vi "HFRR ADV v022 new software.vi"() -> ()   [LabVIEW 2025] (continued)
            n3909 = Index Array(array=w5040, index #1=1 ("index")) -> (element #1=w5039:string, element #2=w5038:string, element #3=w5037:string, element #4=w5036:string, element #5=w5035:string, element #6=w5034:string)  [unwired: 5 in]
            n3910 = Index Array(array=w5030, index #1=1 ("index")) -> (element #1=w5029:string, element #2=w5028:string, element #3=w5027:string, element #4=w5026:string, element #5=w5025:string, element #6=w5024:string)  [unwired: 5 in]
            n3911 = Index Array(array=w5059, index #1=1 ("index")) -> (element #1=w5058:string, element #2=w5057:string, element #3=w5056:string, element #4=w5055:string, element #5=w5045:string, element #6=w5044:string)  [unwired: 5 in]
            n3912 = Index Array(array=w4979, index #1=1 ("index")) -> (element #1=w5011:string, element #2=w5010:string, element #3=w5009:string, element #4=w5008:string, element #5=w5007:string, element #6=w5006:string)  [unwired: 5 in]
            n3913 = local read "SEN.RUN HRS"() -> (w4982:dbl)
            n3914 = Divide(x=w4986, y=w4994) -> (x/y=w4993:dbl)
            n3915 = Increment(x=w4993) -> (x+1=w4989:dbl)
            n3916 = Number To Decimal String(number=w4989) -> (decimal integer string=→"run hrs":string)  [unwired: 1 in]
            n3917 = Divide(x=w4982, y=3600.0 ("f")) -> (x/y=w4977:dbl)
            n3918 = Round To Nearest(number=w4977) -> (nearest integer value=w4975:dbl)
            n3919 = Number To Decimal String(number=w4975) -> (decimal integer string=w4976:string)  [unwired: 1 in]
            n3920 = Number To Decimal String(number=w4984) -> (decimal integer string=w4985:string)  [unwired: 1 in]
            n3921 = local read "Model No"() -> (w4990:string)
            n3922 = local read "UUID"() -> (w5085:string)
            n3923 = local read "Serial No"() -> (w5089:string)
            n3924 = local read "Secret Key"() -> (w5090:string)
            n3925 = Concatenate Strings("\",\"MachineSerialNumber\":\"" ("string"), w5089) -> (w5093:string)
            n3926 = Concatenate Strings("\",\"ModelNumber\":\"" ("string"), w4990) -> (w4991:string)
            n3927 = Concatenate Strings("\",\"MachineRuntimeHours\":\"" ("string"), w4976) -> (w5094:string)
            n3928 = Concatenate Strings("\",\"MachineRuntimeCycles\":\"", w4985) -> (w5087:string)
            n3929 = Concatenate Strings(w5043, w5039) -> (w5073:string)
            n3930 = Concatenate Strings(w5042, w5029) -> (w5074:string)
            n3931 = Concatenate Strings(w5041, w5011) -> (w5072:string)
            n3932 = Concatenate Strings(w5093, w4991, w5094, w5087) -> (w5096:string)
            n3933 = Concatenate Strings(w5043, w5038) -> (w5070:string)
            n3934 = Concatenate Strings(w5042, w5028) -> (w5069:string)
            n3935 = Concatenate Strings(w5041, w5010) -> (w5071:string)
            n3936 = Concatenate Strings(w5043, w5037) -> (w5065:string)
            n3937 = Concatenate Strings(w5042, w5027) -> (w5066:string)
            n3938 = Concatenate Strings(w5041, w5009) -> (w5064:string)
            n3939 = Concatenate Strings(w5043, w5036) -> (w5062:string)
            n3940 = Concatenate Strings(w5042, w5026) -> (w5061:string)
            n3941 = Concatenate Strings(w5041, w5008) -> (w5063:string)
            n3942 = Concatenate Strings(w5073, w5074, w5072) -> (w5075:string)
            n3943 = Concatenate Strings(w5043, w5035) -> (w5052:string)
            n3944 = Concatenate Strings(w5042, w5025) -> (w5053:string)
            n3945 = Concatenate Strings(w5043, w5034) -> (w5049:string)
            n3946 = Concatenate Strings(w5042, w5024) -> (w5048:string)
            n3947 = Concatenate Strings(w5041, w5007) -> (w5051:string)
            n3948 = Concatenate Strings(w5041, w5006) -> (w5050:string)
            n3949 = Concatenate Strings("{\"SecretKey\":\"", w5090, w5096, "\",\"UUID\" : \"", w5085, "\",\"SensorInformation\":", "[{" ("string")) -> (w5023:string)
            n3950 = Concatenate Strings(w5070, w5069, w5071) -> (w5068:string)
            n3951 = Concatenate Strings(w5065, w5066, w5064) -> (w5067:string)
            n3952 = Concatenate Strings(w5062, w5061, w5063) -> (w5060:string)
            n3953 = Concatenate Strings(w5052, w5053, w5051) -> (w5054:string)
            n3954 = Concatenate Strings(w5049, w5048, w5050) -> (w5047:string)
            n3955 = Concatenate Strings(w5046, w5058, w5075, w5016) -> (w5022:string)
            n3956 = Concatenate Strings(w5046, w5057, w5068, w5016) -> (w5021:string)
            n3957 = Concatenate Strings(w5046, w5056, w5067, w5016) -> (w5020:string)
            n3958 = Concatenate Strings(w5046, w5055, w5060, w5016) -> (w5019:string)
            n3959 = Concatenate Strings(w5046, w5045, w5054, w5016) -> (w5018:string)
            n3960 = Concatenate Strings(w5046, w5044, w5047, "\"}" ("string")) -> (w5017:string)
            n3961 = Concatenate Strings(w5023, w5022, w5021, w5020, w5019, w5018, w5017, "]}" ("string")) -> (w5014:string)
            n3962 = local read "SEN.RUN HRS"() -> (w4981:dbl)
            n3963 = disable-structure shown="Disabled" {
              frame Disabled {
                n3964 = local read "state"() -> (w5100:string[])
                n3965 = Delete From Array(array=w5100, index=0) -> (array with subset deleted=w5098:string[])  [unwired: 1 in, 1 out]
                n3966 = for {
                  N: 6 -> [_]
                  tunnel: w5098 -> [w5111] mode=indexing
                  tunnel: [w5110] -> w5097 mode=indexing
                  n3967 = Equal?(x=w5111, y="Warning") -> (x = y?=w5107:bool)
                  n3968 = Equal?(x=w5111, y="Healthy") -> (x = y?=w5104:bool)
                  n3969 = Select(t="2" ("y"), s=w5107, f="3" ("y")) -> (s? t:f=w5102:string)
                  n3970 = Select(t="1" ("y"), s=w5104, f=w5102) -> (s? t:f=w5110:string)
                }
                "state1" <- w5097
              }
              frame Enabled {
              }
            }
            n3971 = stacked-sequence {
              tunnel: w5014 -> [w5122 _ _]
              tunnel: [_ _ w5138] -> _
              frame #0 {
                (unwired) FALSE ("convert eol (F)")
                w5124 = enum16{"start", "end", "current"}."start" ("pos mode (0:2)")
                n3972 = local read "Path"() -> (w5118:path)
                n3973 = Path To String(path=w5118) -> (string=w5130:string)
                n3974 = Concatenate Strings(w5130, "\\", "Sensor File Name") -> (w5131:string)
                n3975 = local write "standard output 2"(" ") -> ()
                n3976 = String To Path(string=w5131) -> (path=w5121:path)
                n3977 = call <vilib>:"Open_Create_Replace File.vi"("advisory dialog? (display:T)"=FALSE, "function (open:0)"=T32."create or replace", "file path"=w5121) -> ("error out"=w5134:errorcluster, "refnum"=w5133:refnum<file>)  [unwired: 5 in, 2 out]
                n3978 = Set File Position(refnum=w5133, from (0:start)=w5124, error in=w5134) -> (refnum out=w5114:refnum<file>, error out=w5113:errorcluster)  [unwired: 1 in]
                n3979 = Write to Binary File(file (use dialog)=w5114, data=" ", error in=w5113, 5:FALSE ("prepend array or string size? (T)")) -> (refnum out=w5125:refnum<file>, error out=w5126:errorcluster)  [unwired: 2 in, 1 out]
                n3980 = Set File Position(offset (in bytes) (0)=w5124, refnum=w5125, error in=w5126) -> (refnum out=w5117:refnum<file>, error out=w5116:errorcluster)  [unwired: 1 in]
                n3981 = Write to Binary File(file (use dialog)=w5117, data=w5122, error in=w5116, 5:FALSE ("prepend array or string size? (T)")) -> (error out=w5120:errorcluster)  [unwired: 2 in, 2 out]
                n3982 = flat-sequence {
                  tunnel: w5121 -> [w5136]
                  tunnel: w5120 -> [_]
                  frame #0 {
                    n3983 = call <vilib>:"Read Characters From File.vi"("file path (dialog if empty)"=w5136) -> ("character string"=→"Sensor Health JSON string":string)  [unwired: 5 in, 3 out]
                  }
                }
                "SinglePoint  2" <- w5122
              }
              frame #1 {
              }
              frame #2 {
                (unwired) "\"Stored\": true" ("string")
                n3984 = call <vilib>:"System Exec.vi"("run minimized? (F)"=TRUE, "wait until completion? (T)"=TRUE, "working directory"=path "C:/LAB-IQ-NXT", "command line"="C:\\LAB-IQ-NXT\\JPostH.bat") -> ("standard error"=→"Respose From Server 2":string, "standard output"=w5141:string)  [unwired: 4 in, 2 out]
                "standard output 2" <- w5141
                n3985 = Match Pattern(string=w5141, regular expression="JSONH Check String") -> (match substring=w5139:string, offset past match=w5138:i32)  [unwired: 1 in, 2 out]
                n3986 = Equal?(x=w5139, y="JSONH Check String") -> (x = y?=→"Upload \nConfirmed 2":bool)
              }
            }
            n3987 = Divide(x=w4981, y=3600.0 ("f")) -> (x/y=w4974:dbl)
            n3988 = local read "run time"() -> (w5031:string[])
            n3989 = Round To Nearest(number=w4974) -> (nearest integer value=w4973:dbl)
            n3990 = Number To Decimal String(number=w4973) -> (decimal integer string=w4972:string)  [unwired: 1 in]
            n3991 = Index Array(array="Sensor Information", index (col) #1=0 ("disabled index (col)"), index (col) #2=1 ("index (col)"), index (col) #3=2 ("index (col)"), index (col) #4=3 ("index (col)")) -> (element #1=→"Sensor name":string[], element #2=→"model num":string[], element #3=→"run time":string[], element #4=→"state":string[])  [unwired: 4 in]
            n3992 = Insert Into Array(array=w5031, index=1, new element #1=w4972, new element #2=w4972, new element #3=w4972, new element #4=w4972, new element #5=w4972, new element #6=w4972) -> (w4996:string[])
            "run" <- w4996
            n3993 = local read "out"() -> (w4978:string[])
            n3994 = local read "Sensor Information"() -> (w4998:string[][])
            n3995 = Replace Array Subset(array=w4998, new element #1=w4996, index (col) #1=2 ("disabled index (col)"), new element #2=w4978, index (col) #2=3 ("index (col)")) -> (w4997:string[][])  [unwired: 2 in]
            n3996 = local write "Sensor Information"(w4997) -> ()
          }
        }
        n3997 = case shown="True" w4945 {
          frame False {
          }
          frame True {
            n3998 = Equal?(x="FLAG", y=0.0) -> (x = y?=w4962:bool)
            n3999 = case shown="False" w4962 {
              frame False {
                n4000 = Get Date/Time In Seconds() -> (seconds since 1Jan1904=w4968:timestamp)
                n4001 = local read "START 2"() -> (w4966:dbl)
                n4002 = To Double Precision Float(number=w4968) -> (double precision float=w4967:dbl)
                n4003 = Subtract(x=w4967, y=w4966) -> (x-y=→"SENSOR TIME  2":dbl)
              }
              frame True {
                n4004 = Get Date/Time In Seconds() -> (seconds since 1Jan1904=w4970:timestamp)
                n4005 = To Double Precision Float(number=w4970) -> (double precision float=→"START 2":dbl)
                n4006 = local write "FLAG"(100.0 ("FLAG")) -> ()
              }
            }
          }
        }
        n4007 = disable-structure shown="Disabled" {
          disable-tunnel: w4948 -> [w4957 _]
          disable-tunnel: [w4956 _] -> w4947
          frame Disabled {
            n4008 = local read "Json St Flg"() -> (w4955:bool)
            n4009 = case shown="True" w4955 {
              tunnel: w4957 -> [w4958 w4960]
              tunnel: [w4958 w4959] -> w4956
              frame False {
              }
              frame True {
                n4010 = Increment(x=w4960) -> (x+1=w4959:dbl)
                "T cycle" <- w4959
                n4011 = local write "Json St Flg"(FALSE ("Json St Flg")) -> ()
              }
            }
          }
          frame Enabled {
          }
        }
        n4012 = local read "Quit"() -> (w4942:bool)
      }
    }
    frame Enabled {
    }
  }
  n4013 = stacked-sequence {
    tunnel: [w5340] -> w44
    frame #0 {
      w5340 = FALSE ("Upload \nConfirmed")
      n4014 = local write "Upload \nConfirmed"(w5340) -> ()
      n4015 = local write "St Str"("") -> ()
    }
  }
  n4016 = disable-structure shown="Disabled" {
    disable-tunnel: w44 -> [w5341 _]
    frame Disabled {
      n4017 = case shown="True" {
        selector: _ -> [_ _]
        tunnel: w5341 -> [_ w5342]
        frame False {
        }
        frame True {
          n4018 = while {
            tunnel: [w5348] -> _
            tunnel: w5342 -> [_]
            i -> [w5348]
            stop <- w5343 stop-if-true
            n4019 = local read "Json End Flg"() -> (w5347:bool)
            n4020 = Wait (ms)(milliseconds to wait=u32 20 ("Refresh Rate (ms)")) -> ()  [unwired: 1 out]
            n4021 = local read "refresh flag"() -> (w5344:bool)
            n4022 = local read "RUN"() -> (w5345:bool)
            n4023 = And(x=w5345, y=w5344) -> (x .and. y?=w5346:bool)
            n4024 = Or(x=w5346, y=w5347) -> (x .or. y?=w5349:bool)
            "AR Led" <- w5349
            n4025 = case shown="True" w5349 {
              frame False {
              }
              frame True {
                w5366 = "\",\""
                n4026 = local read "UUID"() -> (w5364:string)
                n4027 = local write "refresh flag"(FALSE ("refresh flag")) -> ()
                n4028 = local read "time"() -> (w5353:dbl)
                n4029 = Multiply(x=w5353, y=60.0) -> (x*y=w5352:dbl)
                n4030 = Concatenate Strings("UUID\" : \"", w5364, "\"}") -> (w5367:string)
                n4031 = Number To Fractional String(number=w5352, width (-)=i16 10, precision (6)=i16 4) -> (F-format string=w5381:string)  [unwired: 1 in]
                n4032 = Concatenate Strings("{", "\"Time\":\"", w5381, w5366) -> (w5376:string)
                n4033 = stacked-sequence {
                  tunnel: w5366 -> [w5429 w5437 w5444 w5452 w5460 w5469 w5476]
                  tunnel: [w5430 _ _ _ _ _ _] -> w5380
                  tunnel: [_ w5438 _ _ _ _ _] -> w5379
                  tunnel: [_ _ w5445 _ _ _ _] -> w5378
                  tunnel: [_ _ _ w5454 _ _ _] -> w5377
                  tunnel: w5367 -> [_ _ _ _ _ _ w5487]
                  tunnel: [_ _ _ _ _ _ w5486] -> w5363
                  tunnel: [_ _ _ _ _ w5466 _] -> w5362
                  tunnel: [_ _ _ _ w5459 _ _] -> w5361
                  frame #0 {
                    n4034 = local read "NORMAL LOAD"() -> (w5428:dbl)
                    n4035 = Number To Fractional String(number=w5428, width (-)=i16 10, precision (6)=i16 4) -> (F-format string=w5431:string)  [unwired: 1 in]
                    n4036 = Concatenate Strings("NormalLoad\":\"", w5431, w5429) -> (w5430:string)
                  }
                  frame #1 {
                    n4037 = local read "Temp"() -> (w5436:dbl)
                    n4038 = Number To Fractional String(number=w5436, width (-)=i16 10, precision (6)=i16 4) -> (F-format string=w5439:string)  [unwired: 1 in]
                    n4039 = Concatenate Strings("Temperature\":\"", w5439, w5437) -> (w5438:string)
                  }
                  frame #2 {
                    n4040 = local read "cof"() -> (w5442:dbl)
                    n4041 = Number To Fractional String(number=w5442, width (-)=i16 10, precision (6)=i16 4) -> (F-format string=w5446:string)  [unwired: 1 in]
                    n4042 = Concatenate Strings("FrictionalForce\":\"", w5446, w5444) -> (w5445:string)
                  }
                  frame #3 {
                    n4043 = local read "Set Hz"() -> (w5450:dbl)
                    n4044 = Multiply(x=w5450, y=60.0) -> (x*y=w5449:dbl)
                    n4045 = Number To Fractional String(number=w5449, width (-)=i16 10, precision (6)=i16 4) -> (F-format string=w5455:string)  [unwired: 1 in]
                    n4046 = Concatenate Strings("Speed\":\"", w5455, w5452) -> (w5454:string)
                  }
                  frame #4 {
                    n4047 = local read item#-1() -> (w5458)
                    n4048 = Number To Fractional String(number=w5458, width (-)=i16 10, precision (6)=i16 4) -> (F-format string=w5462:string)  [unwired: 1 in]
                    n4049 = Concatenate Strings("LinearDeformation\":\"", w5462, w5460) -> (w5459:string)
                  }
                  frame #5 {
                    n4050 = local read "AIR TEMP"() -> (w5465:dbl)
                    n4051 = local read "Json St Flg"() -> (w5467:bool)
                    n4052 = local read "Json End Flg"() -> (w5468:bool)
                    n4053 = Number To Fractional String(number=w5465, width (-)=i16 10, precision (6)=i16 4) -> (F-format string=w5471:string)  [unwired: 1 in]
                    n4054 = Concatenate Strings("Vibration\":\"", w5471, w5469) -> (w5466:string)
                    n4055 = And(x=w5467, y=w5468) -> ()  [unwired: 1 out]
                  }
                  frame #6 {
                    n4056 = local read "Json End Flg"() -> (w5475:bool)
                    n4057 = Get Date/Time In Seconds() -> (seconds since 1Jan1904=w5483:timestamp)
                    n4058 = local read "Json St Flg"() -> (w5474:bool)
                    n4059 = To Double Precision Float(number=w5483) -> (double precision float=w5482:dbl)
                    n4060 = Subtract(x=w5482, y=2082844800.0) -> (x-y=w5480:dbl)
                    n4061 = Number To Fractional String(number=w5480, width (-)=i16 12, precision (6)=i16 0) -> (F-format string=w5477:string)  [unwired: 1 in]
                    n4062 = case shown="True" w5475 {
                      tunnel: ["" w5490] -> w5484
                      tunnel: w5477 -> [_ w5491]
                      tunnel: w5476 -> [_ w5489]
                      frame False {
                      }
                      frame True {
                        n4063 = local write "Json End Flg"(FALSE ("Json St Flg")) -> ()
                        n4064 = Concatenate Strings("End\": \"", w5491, w5489) -> (w5490:string)
                      }
                    }
                    n4065 = case shown="True" w5474 {
                      tunnel: [w5494 w5497] -> w5485
                      tunnel: w5477 -> [_ w5498]
                      tunnel: w5476 -> [_ w5495]
                      frame False {
                        n4066 = local read "St Str"() -> (w5494:string)
                      }
                      frame True {
                        n4067 = Concatenate Strings("Start\":\"", w5498, w5495) -> (w5497:string)
                        "St Str" <- w5497
                        n4068 = local write "Json St Flg"(FALSE ("Json St Flg")) -> ()
                      }
                    }
                    n4069 = Concatenate Strings(w5485, w5484, w5487) -> (w5486:string)
                  }
                }
                n4070 = local read "FILE"() -> (w5355:string)
                n4071 = Concatenate Strings("\",\"OperatorID\":\"" ("string"), "Operator ID") -> (w5358:string)
                n4072 = Concatenate Strings("\",\"DatasetTitle\":\"" ("string"), w5355) -> (w5357:string)
                n4073 = Concatenate Strings("\",\"SerialNumber\":\"" ("string"), "Serial No") -> (w5387:string)
                n4074 = Concatenate Strings("\",\"ModelNumber\":\"" ("string"), "Model No") -> (w5386:string)
                n4075 = Concatenate Strings(w5387, w5386) -> (w5369:string)
                n4076 = Concatenate Strings("{\"SecretKey\":\"", "Secret Key", w5369, w5358, w5357, "\",\"Samples\":[") -> (w5374:string)
                n4077 = Concatenate Strings(w5376, w5380, w5379, w5378, w5377, w5361, w5362, w5363) -> (w5375:string)
                n4078 = Concatenate Strings(w5374, w5375, "]}") -> (w5373:string)
                n4079 = stacked-sequence {
                  tunnel: w5373 -> [w5402 _ _]
                  tunnel: [_ _ w5419] -> _
                  frame #0 {
                    (unwired) FALSE ("convert eol (F)")
                    w5404 = enum16{"start", "end", "current"}."start" ("pos mode (0:2)")
                    n4080 = Path To String(path="Path") -> (string=w5410:string)
                    n4081 = Concatenate Strings(w5410, "\\", "Data File Name") -> (w5412:string)
                    n4082 = local write "standard output"(" ") -> ()
                    n4083 = String To Path(string=w5412) -> (path=w5401:path)
                    n4084 = call <vilib>:"Open_Create_Replace File.vi"("advisory dialog? (display:T)"=FALSE, "function (open:0)"=T32."create or replace", "file path"=w5401) -> ("error out"=w5415:errorcluster, "refnum"=w5414:refnum<file>)  [unwired: 5 in, 2 out]
                    n4085 = Set File Position(refnum=w5414, from (0:start)=w5404, error in=w5415) -> (refnum out=w5395:refnum<file>, error out=w5394:errorcluster)  [unwired: 1 in]
                    n4086 = Write to Binary File(file (use dialog)=w5395, data=" ", error in=w5394, 5:FALSE ("prepend array or string size? (T)")) -> (refnum out=w5405:refnum<file>, error out=w5406:errorcluster)  [unwired: 2 in, 1 out]
                    n4087 = Set File Position(offset (in bytes) (0)=w5404, refnum=w5405, error in=w5406) -> (refnum out=w5398:refnum<file>, error out=w5397:errorcluster)  [unwired: 1 in]
                    n4088 = Write to Binary File(file (use dialog)=w5398, data=w5402, error in=w5397, 5:FALSE ("prepend array or string size? (T)")) -> (error out=w5400:errorcluster)  [unwired: 2 in, 2 out]
                    n4089 = flat-sequence {
                      tunnel: w5401 -> [w5417]
                      tunnel: w5400 -> [_]
                      frame #0 {
                        n4090 = call <vilib>:"Read Characters From File.vi"("file path (dialog if empty)"=w5417) -> ("character string"=→"JSON string":string)  [unwired: 5 in, 3 out]
                      }
                    }
                    "SinglePoint" <- w5402
                  }
                  frame #1 {
                  }
                  frame #2 {
                    (unwired) "\"Stored\": true" ("string")
                    n4091 = call <vilib>:"System Exec.vi"("run minimized? (F)"=TRUE, "wait until completion? (T)"=TRUE, "working directory"=path "C:/LAB-IQ-NXT", "command line"="C:\\LAB-IQ-NXT\\JPost.bat") -> ("standard error"=→"Respose From Server":string, "standard output"=w5422:string)  [unwired: 4 in, 2 out]
                    "standard output" <- w5422
                    n4092 = Match Pattern(string=w5422, regular expression="JSON Check String") -> (match substring=w5420:string, offset past match=w5419:i32)  [unwired: 1 in, 2 out]
                    n4093 = Equal?(x=w5420, y="JSON Check String") -> (x = y?=→"Upload \nConfirmed":bool)
                  }
                }
              }
            }
            n4094 = local read "Quit"() -> (w5343:bool)
          }
        }
      }
    }
    frame Enabled {
    }
  }
  n4095 = disable-structure shown="Disabled" {
    disable-tunnel: _ -> [w5505 _]
    frame Disabled {
      n4096 = while {
        shift-right: [w5513] -> w5501
        shift-left: _ -> [w5514]
        shift-right: [w5511] -> w5502
        shift-left: errorcluster {"status"=TRUE, "code"=0, "source"="Init"} ("error out") -> [w5512]
        shift-right: [w5509] -> _
        shift-left: "" -> [w5510]
        tunnel: [w5507] -> _
        tunnel: w5505 -> [_]
        i -> [w5507]
        stop <- w5506 stop-if-true
        n4097 = flat-sequence {
          tunnel: [w5515] -> w5508
          frame #0 {
            n4098 = Wait (ms)(milliseconds to wait=10.0 ("Delay")) -> (millisecond timer value=w5515:u32)
          }
        }
        n4099 = case shown="No Error" w5512 {
          selector: w5512 -> [w5545 w5664]
          tunnel: [w5528 w5666] -> w5513
          tunnel: [w5527 w5665] -> w5511
          tunnel: w5514 -> [w5546 w5658]
          tunnel: w5510 -> [w5526 w5657]
          tunnel: [w5525 w5657] -> w5509
          tunnel: w5508 -> [_ _]
          frame No Error {
            n4100 = Concatenate Strings("\r", "\n") -> (w5537:string)  [unwired: 1 in]
            n4101 = case shown="True" w5538 {
              tunnel: w5546 -> [w5570 w5577]
              tunnel: w5545 -> [w5569 w5576]
              tunnel: [w5570 w5575] -> w5544
              tunnel: [w5569 w5574] -> w5524
              tunnel: w5537 -> [_ w5573]
              frame False {
              }
              frame True {
                n4102 = VISA Write(VISA resource name=w5577, write buffer=w5573, error in (no error)=w5576) -> (VISA resource name out=w5575:refnum<visa-resource-name>, error out=w5574:errorcluster)  [unwired: 1 out]
                n4103 = local write "Read String"("") -> ()
                n4104 = local write item#-1(FALSE) -> ()
              }
            }
            n4105 = property class="Instr"(reference=w5544, error in=w5524) -> (reference out=w5543:refnum<visa-resource-name>, error out=w5542:errorcluster, "Serial Settings:Number of Bytes at Serial Port"=w5541:u32)
            n4106 = Greater?(x=w5541, y=u32 100) -> (0:w5539:bool)
            n4107 = case shown="True" w5539 {
              tunnel: w5543 -> [w5580 w5604]
              tunnel: w5542 -> [w5579 w5603]
              tunnel: w5541 -> [_ w5602]
              tunnel: [w5580 w5601] -> w5530
              tunnel: [w5579 w5600] -> w5529
              tunnel: w5526 -> [w5578 w5599]
              tunnel: [w5578 ""] -> w5525
              frame False {
              }
              frame True {
                w5589 = u32 6 ("y")
                # "Page 84 of \nmanual"
                n4108 = VISA Read(VISA resource name=w5604, byte count=w5602, error in (no error)=w5603) -> (VISA resource name out=w5601:refnum<visa-resource-name>, read buffer=w5597:string, error out=w5600:errorcluster)  [unwired: 1 out]
                n4109 = while {
                  tunnel: w5597 -> [w5653]
                  tunnel: [w5649] -> w5591 mode=indexing
                  tunnel: [w5643] -> w5595 mode=indexing
                  tunnel: [w5641] -> _
                  i -> [w5641]
                  stop <- w5646 stop-if-true
                  n4110 = String Subset(string=w5653, offset (0)=w5641) -> (substring=w5648:string)  [unwired: 1 in]
                  n4111 = String To Byte Array(string=w5648) -> (unsigned byte array=w5652:u8[])
                  n4112 = String Length(string=w5648) -> (length=w5647:i32)
                  n4113 = Index Array(array=w5652) -> (element=w5651:u8)  [unwired: 1 in]
                  n4114 = Equal To 0?(x=w5647) -> (x = 0?=w5646:bool)
                  n4115 = Number To Boolean Array(number=w5651) -> (Boolean array=w5645:bool[])
                  n4116 = Reverse 1D Array(array=w5645) -> (reversed array=w5644:bool[])
                  n4117 = And(x=w5645, y=bool[] [FALSE, FALSE, FALSE, FALSE, FALSE, FALSE, TRUE, TRUE] ("Boolean array")) -> (x .and. y?=w5649:bool[])
                  n4118 = And(x=w5644, y=bool[] [FALSE, FALSE, TRUE, TRUE, TRUE, TRUE, TRUE, TRUE] ("Boolean array")) -> (x .and. y?=w5643:bool[])
                }
                n4119 = Concatenate Strings(w5599, w5597) -> (→"Read String":string)
                n4120 = while {
                  tunnel: w5591 -> [w5640] mode=indexing
                  tunnel: [w5636] -> w5594
                  i -> [w5636]
                  stop <- w5637 stop-if-true
                  n4121 = Search 1D Array(1D array=w5640, element=TRUE) -> (index of element=w5638:i32)  [unwired: 1 in]
                  n4122 = Less Than 0?(x=w5638) -> (x < 0?=w5637:bool)
                }
                n4123 = Delete From Array(array=w5595, length=w5594, index (row)=0) -> (array with subset deleted=w5590:bool[][])  [unwired: 1 in, 1 out]
                n4124 = Array Size(array=w5590) -> (size(s)=w5592:i32[])
                n4125 = Index Array(array=w5592) -> (element=w5584:i32)  [unwired: 1 in]
                n4126 = Greater?(x=w5584, y=w5589) -> (0:w5587:bool)
                n4127 = Subtract(x=w5584, y=w5589) -> (x-y=w5588:u32)
                n4128 = Select(t=w5588, s=w5587, f=u32 0) -> (s? t:f=w5585:u32)
                n4129 = while {
                  tunnel: w5590 -> [w5623]
                  tunnel: [w5625] -> w5583 mode=indexing
                  tunnel: w5585 -> [w5607]
                  i -> [w5624]
                  stop <- w5622 stop-if-true
                  w5614 = 6 ("index")
                  w5613 = 2 ("length")
                  # "Page 65 of \nmanual"
                  n4130 = Multiply(x=u32 3 ("y"), y=w5624) -> (x*y=w5621:u32)
                  n4131 = Divide(x=u32 102 ("y"), y=u32 65520) -> (x/y=w5631:dbl)
                  n4132 = Greater Or Equal?(x=w5621, y=w5607) -> (x >= y?=w5622:bool)
                  n4133 = Index Array(array=w5623, index (row) #1=w5621) -> (element #1=w5619:bool[], element #2=w5618:bool[], element #3=w5617:bool[])  [unwired: 5 in]
                  n4134 = Reverse 1D Array(array=w5619) -> (reversed array=w5612:bool[])
                  n4135 = Reverse 1D Array(array=w5618) -> (reversed array=w5616:bool[])
                  n4136 = Reverse 1D Array(array=w5617) -> (reversed array=w5615:bool[])
                  n4137 = Delete From Array(array=w5612, length=w5613, index=w5614) -> (array with subset deleted=w5608:bool[])  [unwired: 1 out]
                  n4138 = Delete From Array(array=w5616, length=w5613, index=w5614) -> (array with subset deleted=w5609:bool[])  [unwired: 1 out]
                  n4139 = Delete From Array(array=w5615, length=w5613, index=w5614) -> (array with subset deleted=w5610:bool[])  [unwired: 1 out]
                  n4140 = Insert Into Array(array=bool[] [] ("Boolean array"), new element #1=w5608, new element #2=w5609, new element #3=w5610) -> (w5611:bool[])  [unwired: 1 in]
                  n4141 = Boolean Array To Number(Boolean array=w5611) -> (number=w5620:u32)
                  n4142 = Multiply(x=w5631, y=w5620) -> (x*y=w5630:dbl)
                  n4143 = Decrement(x=w5630) -> (x-1=w5629:dbl)
                  n4144 = Divide(x=w5629, y=u32 100) -> (x/y=w5627:dbl)
                  n4145 = Multiply(x=w5627, y=u32 10) -> (x*y=w5625:dbl)
                }
                n4146 = Delete From Array(array=w5583) -> (array with subset deleted=w5582:dbl[])  [unwired: 2 in, 1 out]
                "Waveform Graph 5" <- w5582
                "Waveform Chart 3" <- w5582
                n4147 = call-poly <vilib>:"Mean.vi"("X"=w5582) -> ("mean"=w5581:dbl)  [unwired: 1 out]
                n4148 = case shown="True" {
                  selector: _ -> [_ _]
                  tunnel: w5581 -> [_ w5606]
                  frame False {
                  }
                  frame True {
                    n4149 = local write item#-1(FALSE ("Zero 4")) -> ()
                    "z_measure" <- w5606
                  }
                }
              }
            }
            n4150 = local read item#-1() -> (w5521)
            n4151 = local read item#-1() -> (w5520)
            n4152 = local read item#-1() -> (w5522)
            n4153 = local read item#-1() -> (w5519)
            n4154 = case shown="True" w5517 {
              tunnel: w5521 -> [_ w5549]
              tunnel: w5522 -> [_ w5548]
              frame False {
              }
              frame True {
                n4155 = Build Array(w5549, w5548) -> (w5547:void[])
                n4156 = local read item#-1() -> (w5552)
                n4157 = Build Array (concatenate)(w5552, w5547) -> (w5550:void[])
                n4158 = local write item#-1(w5550) -> ()
                n4159 = local write item#-1(FALSE ("Boolean 8")) -> ()
              }
            }
            n4160 = call "Build XY Graph"("Enable"=w5519, "Reset"=w5520, "Y Input"=w5522, "X Input"=w5521) -> ("XY Graph"=w5518:cluster{"Y":dbl[], "Y":dbl[]}[])  [unwired: 6 in, 1 out]
            n4161 = case shown="True" {
              selector: _ -> [_ _]
              frame False {
              }
              frame True {
                n4162 = local read item#-1() -> (w5553)
                n4163 = Index Array(array=w5553, index (col) #1=0 ("disabled index (col)"), index (col) #2=1 ("index (col)")) -> (element #1=w5555, element #2=w5554)  [unwired: 2 in]
                n4164 = call <vilib>:"Linear Fit.vi"("Y"=w5555, "X"=w5554) -> ()  [unwired: 9 in, 5 out]
                n4165 = local write item#-1(FALSE ("Boolean 9")) -> ()
              }
            }
            n4166 = case shown="True" {
              selector: _ -> [_ _]
              frame False {
              }
              frame True {
                n4167 = local write item#-1(dbl[][] [] ("Captured Values")) -> ()
                n4168 = local write item#-1(FALSE ("Boolean 7")) -> ()
              }
            }
            n4169 = Concatenate Strings("\r", "\n") -> (w5532:string, w5531:string)
            n4170 = case shown="True" w5523 {
              tunnel: w5530 -> [w5562 w5568]
              tunnel: w5529 -> [w5561 w5567]
              tunnel: [w5562 w5566] -> w5528
              tunnel: [w5561 w5565] -> w5527
              tunnel: w5532 -> [_ w5564]
              frame False {
              }
              frame True {
                n4171 = VISA Write(VISA resource name=w5568, write buffer=w5564, error in (no error)=w5567) -> (VISA resource name out=w5566:refnum<visa-resource-name>, error out=w5565:errorcluster)  [unwired: 1 out]
                n4172 = local write item#-1(FALSE ("WRITE")) -> ()
              }
            }
          }
          frame Error {
            w5656 = u16 10 items=["1.0"=10, "1.5"=15, "2.0"=20] ("stop bits (10: 1 bit)")
            n4173 = Wait (ms)(milliseconds to wait=u32 20) -> ()  [unwired: 1 out]
            n4174 = VISA Close(VISA resource name=w5658, error in (no error)=w5664) -> (error out=w5663:errorcluster)
            n4175 = call <vilib>:"Clear Errors.vi"("error in (no error)"=w5663) -> ("error out"=w5662:errorcluster)  [unwired: 5 in, 1 out]
            n4176 = call-poly "VISA Configure Serial Port"("timeout (10sec)"=u32 200, "Enable Termination\nChar (T)"=TRUE ("Enable Termination\nChar (T)"), "baud rate (9600)"=u32 921600, "error in (no error)"=w5662, "stop bits (10: 1 bit)"=w5656) -> ("VISA resource name"=w5654:refnum<visa-resource-name>, "VISA resource name out"=w5666:refnum<visa-resource-name>, "error out"=w5665:errorcluster)  [unwired: 8 in]
          }
        }
        n4177 = local read "Quit"() -> (w5506:bool)
      }
      n4178 = VISA Close(VISA resource name=w5501, error in (no error)=w5502) -> (error out=w5500:errorcluster)
      n4179 = call <vilib>:"Clear Errors.vi"("error in (no error)"=w5500) -> ()  [unwired: 5 in, 2 out]
    }
    frame Enabled {
    }
  }
  n4180 = disable-structure shown="Disabled" {
    disable-tunnel: _ -> [w5671 _]
    frame Disabled {
      n4181 = while {
        tunnel: [w5678] -> _
        shift-right: [w5675] -> w5668
        shift-left: _ -> [w5677]
        shift-right: [w5676] -> w5669
        shift-left: errorcluster {"status"=TRUE, "code"=0, "source"="Init"} ("error out") -> [w5674]
        tunnel: w5671 -> [_]
        i -> [w5678]
        stop <- w5672 stop-if-true
        n4182 = flat-sequence {
          tunnel: w5674 -> [w5769]
          tunnel: [w5769] -> w5673
          frame #0 {
            n4183 = Wait (ms)(milliseconds to wait=u32 50) -> ()  [unwired: 1 out]
          }
        }
        n4184 = case shown="No Error" w5673 {
          selector: w5673 -> [w5719 w5762]
          tunnel: w5677 -> [w5718 w5761]
          tunnel: [w5685 w5752] -> w5676
          tunnel: [w5686 w5760] -> w5675
          frame No Error {
            w5712 = T33 {"Mode"=enum."RTU", "Slave Address"=1} ("Serial Parameters")
            n4185 = call-poly <vilib>:"MB Serial Master Query (poly).vi"("VISA resource name"=w5718, "Starting Address"=i16 1000, "Quantity"=u16 1, "Timeout"=u32 1000, "error in"=w5719, "Serial Parameters"=w5712) -> ("VISA resource name out"=w5713:refnum<visa-resource-name>, "Input Registers"=w5715:u16[], "error out"=w5711:errorcluster)  [unwired: 10 in, 1 out]
            n4186 = Random Number (0-1)() -> (number: 0 to 1=w5700:dbl)
            n4187 = Index Array(array=w5715, index=0) -> (element=w5710:u16)
            n4188 = Subtract(x=w5700, y=0.5) -> (x-y=w5699:dbl)
            n4189 = Divide(x=w5710, y=10 ("index")) -> (x/y=w5704:dbl)
            n4190 = Multiply(x=w5699, y=0.5) -> (x*y=w5698:dbl)
            n4191 = Add(x=w5704, y=w5698) -> (x+y=w5703:dbl)
            n4192 = local read "Amb temp"() -> (w5687:dbl)
            n4193 = Multiply(x=w5703, y=0.2) -> (x*y=w5707:dbl)
            n4194 = Multiply(x=w5687, y=0.8) -> (x*y=w5705:dbl)
            n4195 = Add(x=w5707, y=w5705) -> (x+y=w5688:dbl)
            n4196 = local read "set temp old"() -> (w5682:dbl)
            n4197 = local write "Amb temp"(w5688) -> ()
            n4198 = Select(t="SetTemp 2", s="Heater", f=100.0) -> (s? t:f=w5683:dbl)
            n4199 = Not Equal?(x=w5683, y=w5682) -> (x != y?=w5681:bool)
            n4200 = case shown="True" w5681 {
              tunnel: w5713 -> [w5747 w5749]
              tunnel: [w5746 w5749] -> w5693
              tunnel: w5711 -> [w5745 w5748]
              tunnel: [w5744 w5748] -> w5691
              tunnel: w5683 -> [w5739 _]
              tunnel: w5712 -> [w5741 w5750]
              tunnel: [w5741 w5750] -> w5694
              frame True {
                n4201 = Multiply(x=w5739, y=10 ("index")) -> (x*y=w5738:dbl)
                n4202 = call-poly <vilib>:"MB Serial Master Query (poly).vi"("VISA resource name"=w5747, "Address"=u16 0, "Holding Register"=w5738, "Timeout"=u32 1000, "error in"=w5745, "Serial Parameters"=w5741) -> ("VISA resource name out"=w5746:refnum<visa-resource-name>, "error out"=w5744:errorcluster)  [unwired: 11 in, 1 out]
                "set temp old" <- w5739
              }
              frame False {
              }
            }
            n4203 = flat-sequence {
              tunnel: [w5720] -> _
              tunnel: [w5720] -> w5690
              tunnel: w5691 -> [w5720]
              frame #0 {
                n4204 = Wait (ms)(milliseconds to wait=u32 100) -> ()  [unwired: 1 out]
              }
            }
            n4205 = call "Elapsed Time12"("Time Target (s)"=2.0, "Auto Reset"=TRUE) -> ("Time has Elapsed"=w5695:bool)  [unwired: 10 in, 7 out]
            n4206 = case shown="True" w5695 {
              tunnel: w5694 -> [w5724 w5737]
              tunnel: [w5724 w5737] -> _
              tunnel: [w5723 w5735] -> w5686
              tunnel: w5693 -> [w5723 w5736]
              tunnel: [w5722 w5733] -> w5685
              tunnel: w5690 -> [w5722 w5734]
              frame False {
              }
              frame True {
                n4207 = call-poly <vilib>:"MB Serial Master Query (poly).vi"("VISA resource name"=w5736, "Starting Address"=i16 1003 ("Addr"), "Quantity"=u16 1, "Timeout"=u32 1000, "error in"=w5734, "Serial Parameters"=w5737) -> ("VISA resource name out"=w5735:refnum<visa-resource-name>, "Input Registers"=w5730:u16[], "error out"=w5733:errorcluster)  [unwired: 10 in, 1 out]
                n4208 = Index Array(array=w5730, index=0) -> (element=w5729:u16)
                n4209 = Divide(x=w5729, y=u16 10) -> (x/y=w5725:dbl)
                n4210 = local write "set temp old"(w5725) -> ()
                n4211 = local write "SetTemp"(w5725) -> ()
              }
            }
            "Error Code" <- w5685
            n4212 = Unbundle(w5685) -> ("status"=→"TK4 status":bool)  [unwired: 2 out]
            "SetTemp" <- "SetTemp 2"
          }
          frame Error {
            w5764 = u16 0 items=["None", "Odd", "Even", "Mark", "Space"] ("Parity")
            w5765 = u16 0 items=["None", "XON/XOFF", "RTS/CTS", "XON/XOFF & RTS/CTS", "DTR/DSR", "XON/XOFF & DTR/DSR"] ("Flow Control")
            n4213 = VISA Clear(VISA resource name=w5761, error in (no error)=w5762) -> (VISA resource name out=w5755:refnum<visa-resource-name>, error out=w5753:errorcluster)
            n4214 = VISA Close(VISA resource name=w5755, error in (no error)=w5753) -> (error out=w5754:errorcluster)
            n4215 = call <vilib>:"Clear Errors.vi"("error in (no error)"=w5754) -> ("error out"=w5763:errorcluster)  [unwired: 5 in, 1 out]
            n4216 = Unbundle By Name(T33 {"Mode"=enum."RTU", "Slave Address"=1} ("input cluster")) -> ("Mode"=w5766:enum16{"RTU", "ASCII"})
            n4217 = call <vilib>:"MB Serial Init.vi"("Timeout"=u32 100, "Flow Control"=w5765, "Mode"=w5766, "error in (no error)"=w5763, "Parity"=w5764, "Baud Rate"=u32 9600, "VISA resource name"="Lubrication System COM Port :") -> ("error out"=w5752:errorcluster, "VISA resource name out"=w5760:refnum<visa-resource-name>)  [unwired: 3 in]
            n4218 = local write "set temp old"(0.0 ("set temp old")) -> ()
            n4219 = Unbundle(w5752) -> ("status"=w5751:bool)  [unwired: 2 out]
            n4220 = case shown="True" w5751 {
              selector: w5751 -> [_ w5768]
              frame False {
              }
              frame True {
                n4221 = local write "TK4 status"(w5768) -> ()
              }
            }
          }
        }
        n4222 = local read "Quit"() -> (w5672:bool)
      }
      n4223 = VISA Close(VISA resource name=w5668, error in (no error)=w5669) -> (error out=w5667:errorcluster)
      n4224 = call <vilib>:"Clear Errors.vi"("error in (no error)"=w5667) -> ()  [unwired: 5 in, 2 out]
    }
    frame Enabled {
    }
  }
